vi "Read Roles.vi"(8 "error in (no error)":errorcluster, 11 "KeeperPlay in":refnum<class "KeeperPlay.lvclass">) -> (0 "error out":errorcluster, 2 "Roles":T1, 3 "KeeperPlay out":refnum<class "KeeperPlay.lvclass">)   [LabVIEW 2023, in "KeeperPlay.lvclass"]
uses:
  KeeperPlay.lvclass
  KeeperRole_class/KeeperRole.lvclass
  KeeperPlay.lvclass/KeeperPlay.ctl
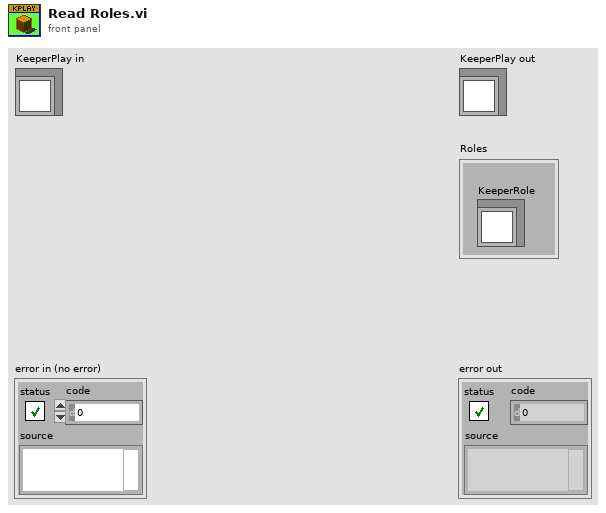
[diagram p1: front panel]
types:
  T1 = cluster{"KeeperRole":refnum<class "KeeperRole.lvclass">}
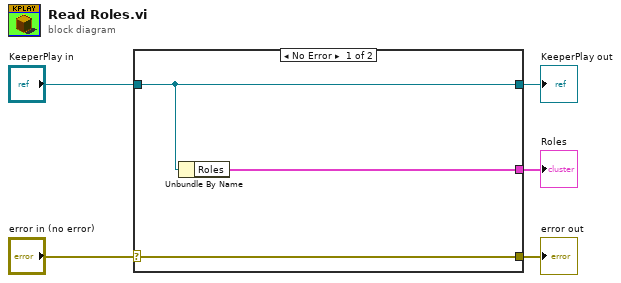
[diagram p0: block diagram]
diagram:
  n1 = case shown="No Error" "error in (no error)" {
    selector: "error in (no error)" -> [w8 w9]
    tunnel: [w8 w9] -> w4
    tunnel: [w7 w10] -> w2
    tunnel: "KeeperPlay in" -> [w7 w10]
    tunnel: [w6 _] -> w1
    frame No Error {
      n2 = Unbundle By Name(w7) -> ("Roles"=w6:T1)
    }
    frame Error {
    }
  }
  "error out" <- w4
  "KeeperPlay out" <- w2
  "Roles" <- w1
